vi "PCO_InitializeLib.vi"(8 "error in (no error)":errorcluster {"code" format="%x"}) -> (0 "error out":errorcluster {"code" format="%x"}, 2 "ErrorMessage":i32 format="%x")   [LabVIEW 2019, in "SDK.lvlib" / "CameraAccess.lvlib"]
doc: "<b>Description:</b>\nThis function is used to set the SC2_cam Library to an initial state. All camera handles have to be closed with PCO_CloseCamera before this function is called.\n\n<b>Supported camera type:</b>\nAll cameras\n\n<b>Descriptor dependency:</b>\nNone"
uses:
  CameraAccess.lvlib
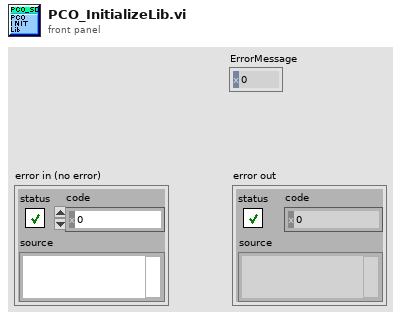
[diagram p1: front panel]
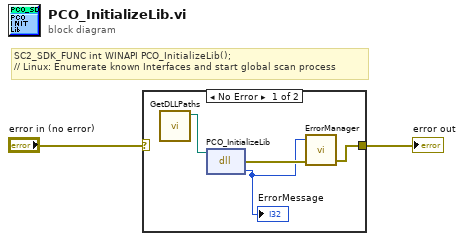
[diagram p0: block diagram]
diagram:
  # "SC2_SDK_FUNC int WINAPI PCO_InitializeLib();\n// Linux: Enumerate known Interfaces and start global scan process"
  n1 = case shown="No Error" "error in (no error)" {
    selector: "error in (no error)" -> [_ w7]
    tunnel: [w6 w7] -> w2
    frame No Error {
      n2 = call "GetDLLPaths.vi"() -> ("SC2_Cam_Path"=w3:path)  [unwired: 8 in, 3 out]
      n3 = dll-call lib="?" fn="PCO_InitializeLib"(path in=w3) -> (error out=w5:errorcluster, "return type"=w4:i32)  [unwired: 2 in, 1 out]
      "ErrorMessage" <- w4
      n4 = call "ErrorManager.vi"("error in (no error)"=w5, "error code"=w4) -> ("error out"=w6:errorcluster)  [unwired: 2 in, 1 out]
    }
    frame Error {
    }
  }
  "error out" <- w2
